vi "nntcpautoa.vi"() -> ()   [LabVIEW 2018, in "nn.lvlib"]
uses:
  nn.lvlib
panel:
  out "Training":bool
  out "resulting string":string
  out "Value":dbl
  out "Output":string
  out "Signal":dynamicdata(graph) caption="Sine"
  out "Class":i32
  in  "Port":u16=54321
  out "error out":errorcluster
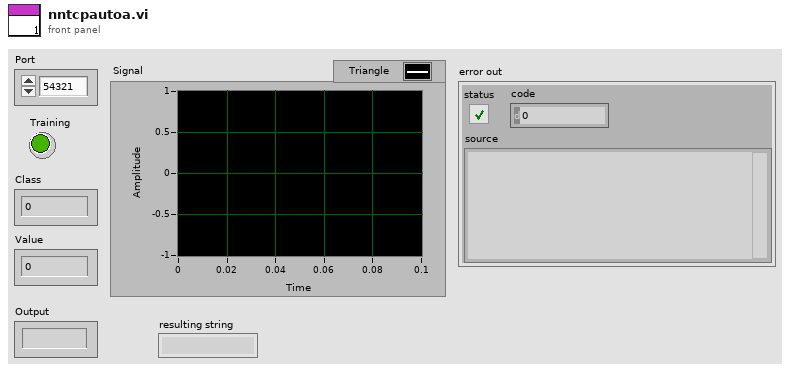
[diagram p1: front panel]
types:
  T1 = enum16{"Standard", "Buffered", "CRLF", "Immediate"}
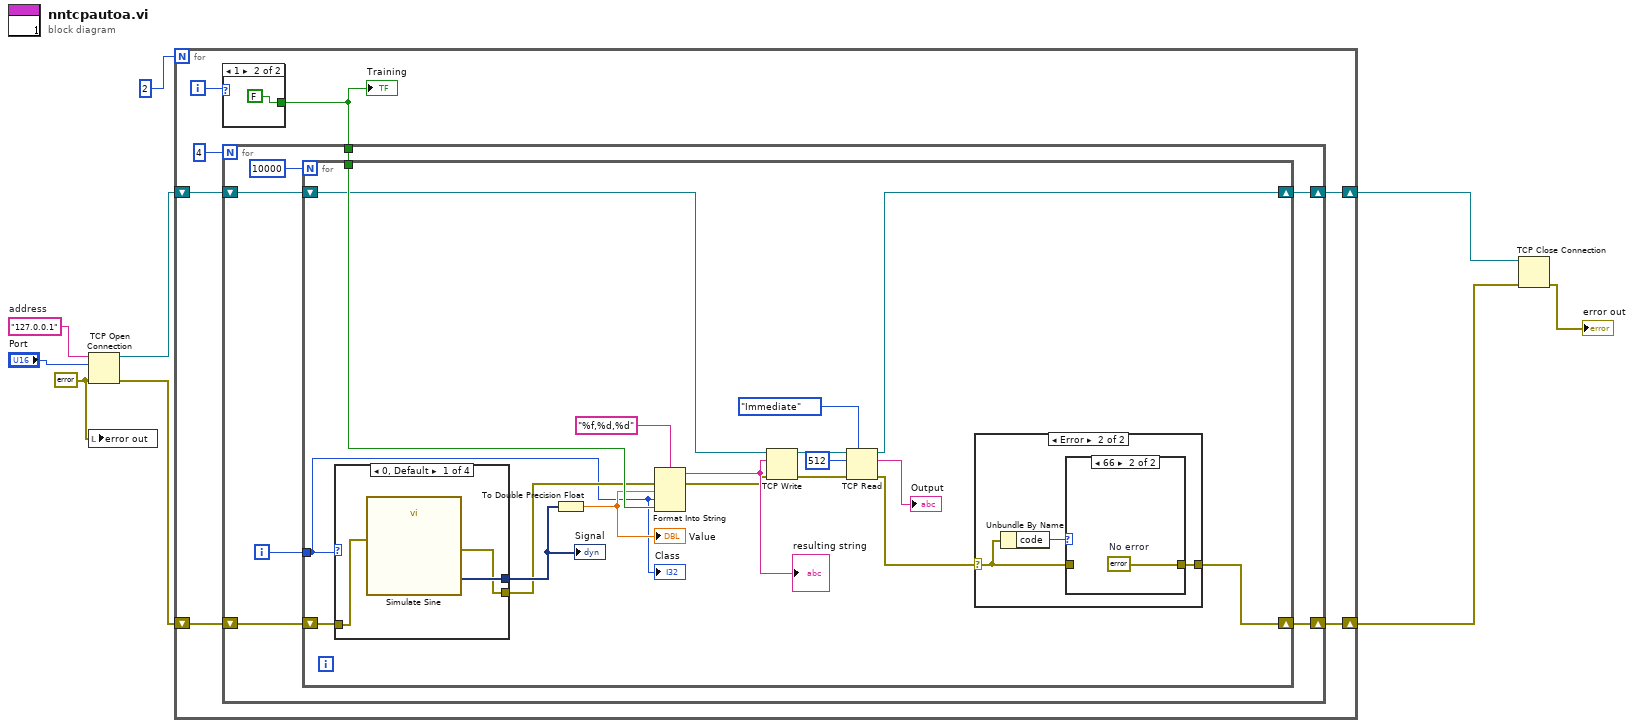
[diagram p0: block diagram]
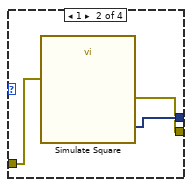
[diagram p4: hidden frame]
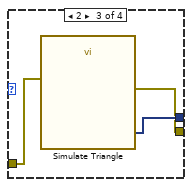
[diagram p5: hidden frame]
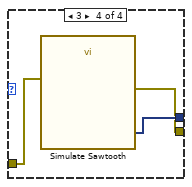
[diagram p6: hidden frame]
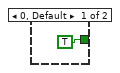
[diagram p7: hidden frame]
diagram:
  w8 = errorcluster {"status"=FALSE, "code"=0, "source"=""} ("error in (no error)")
  w6 = "127.0.0.1"  # address
  n1 = TCP Open Connection(address=w6, remote port or service name="Port", error in (no error)=w8) -> (connection ID=w2:refnum<k5>, error out=w4:errorcluster)  [unwired: 2 in]
  n2 = local write "error out"(w8) -> ()
  n3 = for {
    N: 2 -> [_]
    shift-right: [w13] -> w3
    shift-left: w4 -> [w14]
    shift-right: [w11] -> w1
    shift-left: w2 -> [w12]
    i -> [w16]
    n4 = case shown="1" w16 {
      tunnel: [TRUE FALSE] -> w10
      frame 0, Default {
      }
      frame 1 {
      }
    }
    "Training" <- w10
    n5 = for {
      N: 4 -> [_]
      tunnel: w10 -> [w21]
      shift-right: [w19] -> w13
      shift-left: w14 -> [w20]
      shift-right: [w17] -> w11
      shift-left: w12 -> [w18]
      i -> [w22]
      n6 = for {
        N: 10000 -> [_]
        tunnel: w22 -> [w24]
        tunnel: w21 -> [w40]
        shift-right: [w27] -> w19
        shift-left: w20 -> [w31]
        shift-right: [w29] -> w17
        shift-left: w18 -> [w30]
        n7 = case shown="0, Default" w24 {
          tunnel: [w50 w53 w56 w59] -> w41
          tunnel: [w49 w52 w55 w58] -> w38
          tunnel: w31 -> [w48 w51 w54 w57]
          frame 0, Default {
            n8 = call "Simulate Sine"("error in (no error)"=w48) -> ("Sine"=w50:dynamicdata, "error out"=w49:errorcluster)  [unwired: 13 in]
          }
          frame 1 {
            n9 = call "Simulate Square"("error in (no error)"=w51) -> ("Square"=w53:dynamicdata, "error out"=w52:errorcluster)  [unwired: 13 in]
          }
          frame 2 {
            n10 = call "Simulate Triangle"("error in (no error)"=w54) -> ("Triangle"=w56:dynamicdata, "error out"=w55:errorcluster)  [unwired: 13 in]
          }
          frame 3 {
            n11 = call "Simulate Sawtooth"("error in (no error)"=w57) -> ("Sawtooth"=w59:dynamicdata, "error out"=w58:errorcluster)  [unwired: 13 in]
          }
        }
        "Signal" <- w41
        n12 = To Double Precision Float(number=w41) -> (double precision float=w25:dbl)
        "Value" <- w25
        n13 = Format Into String(format string="%f,%d,%d", error in=w38, w25, w24, w40) -> (resulting string=w33:string, error out=w32:errorcluster)  [unwired: 1 in]
        "resulting string" <- w33
        n14 = TCP Write(connection ID=w30, data in=w33, error in (no error)=w32) -> (connection ID out=w36:refnum<k5>, error out=w37:errorcluster)  [unwired: 1 in, 1 out]
        n15 = TCP Read(connection ID=w36, bytes to read=512, error in (no error)=w37, 7:T1."Immediate" ("mode (standard)")) -> (connection ID out=w29:refnum<k5>, data out=→"Output":string, error out=w28:errorcluster)  [unwired: 1 in]
        n16 = case shown="Error" w28 {
          selector: w28 -> [w42 w44]
          tunnel: [w42 w43] -> w27
          frame No Error {
          }
          frame Error {
            n17 = Unbundle By Name(w44) -> ("code"=w45:i32)
            n18 = case shown="66" w45 {
              tunnel: w44 -> [w46 _]
              tunnel: [w46 w47] -> w43
              frame Default {
              }
              frame 66 {
                w47 = errorcluster {"status"=FALSE, "code"=0, "source"=""}  # No error
              }
            }
          }
        }
        "Class" <- w24
      }
    }
  }
  n19 = TCP Close Connection(connection ID=w1, error in (no error)=w3) -> (error out=→"error out":errorcluster)  [unwired: 1 in, 1 out]
